vi "FlatSecuenceBloqueante.vi"() -> ()   [LabVIEW 2020]
panel:
  out "Boolean 2":bool
  in  "Boolean":bool
  out "Thermometer":dbl(slide) scale=0.0..100.0
  in  "stop":bool
  # "Flat Secuence"
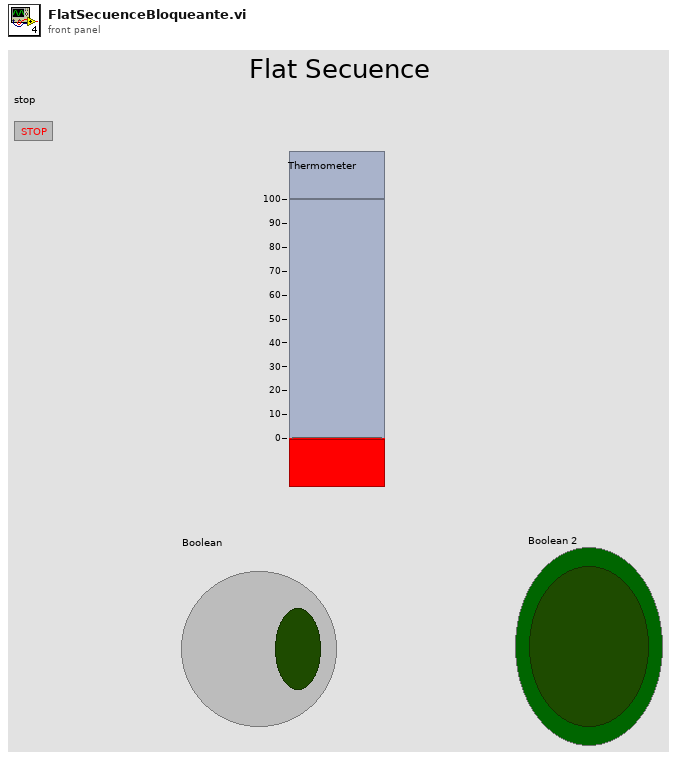
[diagram p1: front panel]
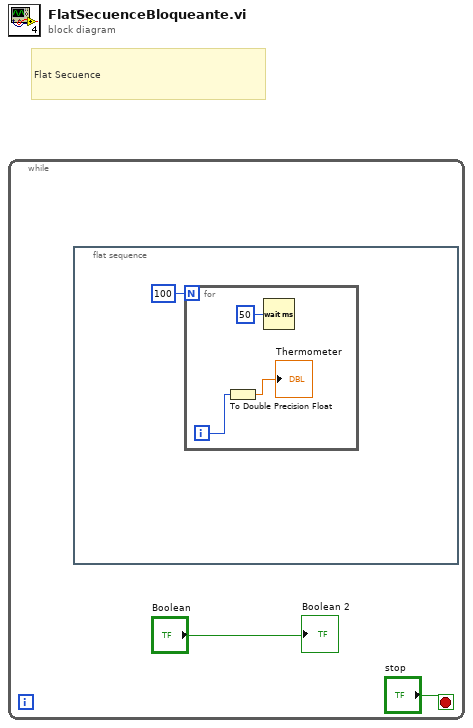
[diagram p0: block diagram]
diagram:
  # "Flat Secuence"
  n1 = while {
    stop <- "stop" stop-if-true
    n2 = flat-sequence {
      frame #0 {
        n3 = for {
          N: 100 -> [_]
          i -> [w5]
          n4 = To Double Precision Float(number=w5) -> (double precision float=→"Thermometer":dbl)
          n5 = Wait (ms)(milliseconds to wait=u32 50) -> ()  [unwired: 1 out]
        }
      }
    }
    "Boolean 2" <- "Boolean"
  }
